vi "ep_Check Part Load Efficiency.vi"(8 "error in (no error)":errorcluster, 10 "full load efficiency [%]":dbl, 11 "additional efficiency information":T1) -> (0 "error out":errorcluster, 3 "efficiency values [%]":dbl[](array[numeric]))   [LabVIEW 2014, in "NI_EP_Motor Monitoring.lvlib"]
uses:
  <vilib>/addons/Electrical Power/Motor Monitoring/NI_EP_Motor Monitoring.lvlib
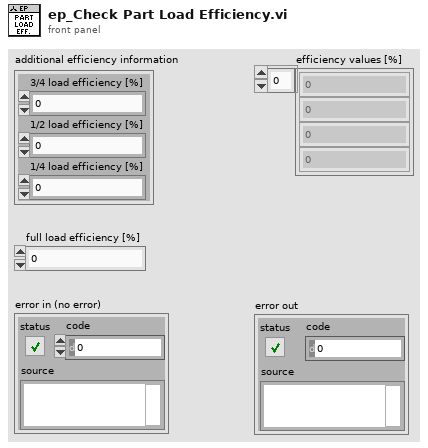
[diagram p1: front panel]
types:
  T1 = cluster{"3/4 load efficiency [%]":dbl, "1/2 load efficiency [%]":dbl, "1/4 load efficiency [%]":dbl}
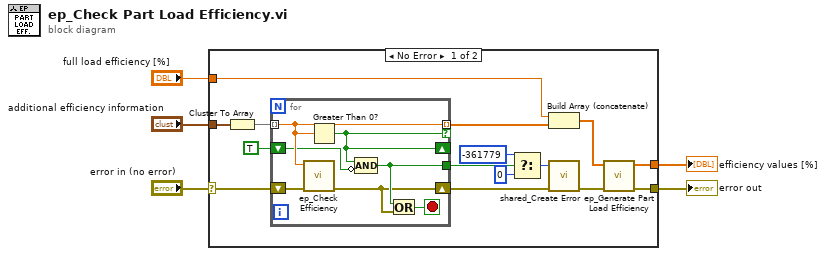
[diagram p0: block diagram]
diagram:
  n1 = case shown="No Error" "error in (no error)" {
    selector: "error in (no error)" -> [w19 w28]
    tunnel: "additional efficiency information" -> [w20 _]
    tunnel: [w9 w28] -> w3
    tunnel: [w8 _] -> w2
    tunnel: "full load efficiency [%]" -> [w11 _]
    frame No Error {
      n2 = Cluster To Array(cluster=w20) -> (array=w14:dbl[])
      n3 = for {
        shift-right: [w21] -> w15
        shift-left: w19 -> [w27]
        tunnel: w14 -> [w26] mode=indexing
        tunnel: [w26] -> w12 mode=indexing if=w25
        shift-right: [w25] -> _
        shift-left: TRUE -> [w24]
        tunnel: [w23] -> w6
        stop <- w22 stop-if-true
        n4 = call <vilib>:"ep_Check Efficiency.vi"("error in (no error)"=w27, "efficiency [%]"=w26) -> ("error out"=w21:errorcluster)  [unwired: 9 in]
        n5 = Greater Than 0?(x=w26) -> (x > 0?=w25:bool)
        n6 = Compound Arithmetic op=AND(w25, invert w24) -> (w23:bool)
        n7 = Or(x=w23, y=w21) -> (x .or. y?=w22:bool)
      }
      n8 = Select(t=-361779, s=w6, f=0 ("error code (0)")) -> (s? t:f=w18:i32)
      n9 = Build Array (concatenate)(w11, w12) -> (w7:dbl[])
      n10 = call <vilib>:"shared_Create Error.vi"("error in (no error)"=w15, "error code (0)"=w18) -> ("error out"=w10:errorcluster)  [unwired: 9 in]
      n11 = call <vilib>:"ep_Generate Part Load Efficiency.vi"("error in (no error)"=w10, "efficiency values in [%]"=w7) -> ("error out"=w9:errorcluster, "efficiency values out [%]"=w8:dbl[])  [unwired: 8 in]
    }
    frame Error {
    }
  }
  "error out" <- w3
  "efficiency values [%]" <- w2
